vi "Main_01B.vi"() -> ()   [LabVIEW 2025]
uses:
  Utility/Universal Utility/TypeDefs_Utility/Cluster_Row-Column.ctl
  9e3f57c0-2ef8-4495-8287-c6a42a5fb955.vi
  Utility/Universal Utility/TypeDefs_Utility/ENUM_4 Directions U-D-L-R.ctl
  Utility/Universal Utility/TypeDefs_Utility/ENUM_8 Directions U-D-L-R.ctl
panel:
  out "count":i32[](array[numeric])
  out "positios":i32[](array[numeric])
  out "Direction Ticks":i32[](array[numeric])
  out "Array":bool[](array[boolean])
  out "MATCH":bool
  in  "Select Data":enum32{"Example", "Puzzle"}(tab)
  in  "Ex Answer":u32=6
  in  "Example":string="L68\nL30\nR48\nL5\nR60\nL55\nL1\nL99\nR14\nL82"
  in  "puzzel Answer":u32=7199
  in  "Puzzle":string="R46\nL11\nR26\nL29\nR14\nL26\nR18\nL38\nL48\nR45\nL8\nL48\nL2\nR34\nR4\nR8\nR35\nR41\nL16\nR31\nL36\nR16\nL22\nL35\nL33\nR42\nR42\nL43\nR28\nL31\nL38\nL47\nL29\nL13\nR13\nL17\nR16\nL20\nL16\nR18\nL21\nR41\nR37\nL10\nR48\nL44\nR26\nR17\nR7\nR78\nL90\nL33\nL91\nR74\nL56\nL53\nL90\nR97\nR42\nR30\nR17\nL47\nR4\nL4\nL23\nR23\nL66\nL45\nL82\nL23\nR90\nR70\nL29\nL66\nR51\nL54\nR54\nR32\nL48\nL95\nL57\nR63\nL14\nR86\nL67\nL45\nL39\nL35\nR19\nR19\nR45\nR87\nR89\nL83\nL57\nR22\nL22\nL36\nL53\nL95\nL616\nL87\nL13\nR67\nR933\nL70\nR75\nR74\nL16\nR20\nR17\nR45\nL92\nL64\nL61\nL28\nR541\nL42\nR1\nR27\nL77\nR850\nR39\nL39\nL373\nR66\nR53\nR16\nL28\nR66\nL7\nL68\nR355\nL80\nR52\nR48\nL16\nR13\nR78\nR330\nR995\nR57\nR643\nR31\nL26\nL1\nR96\nL93\nL48\nL59\nR..."
  out "Answer":u32
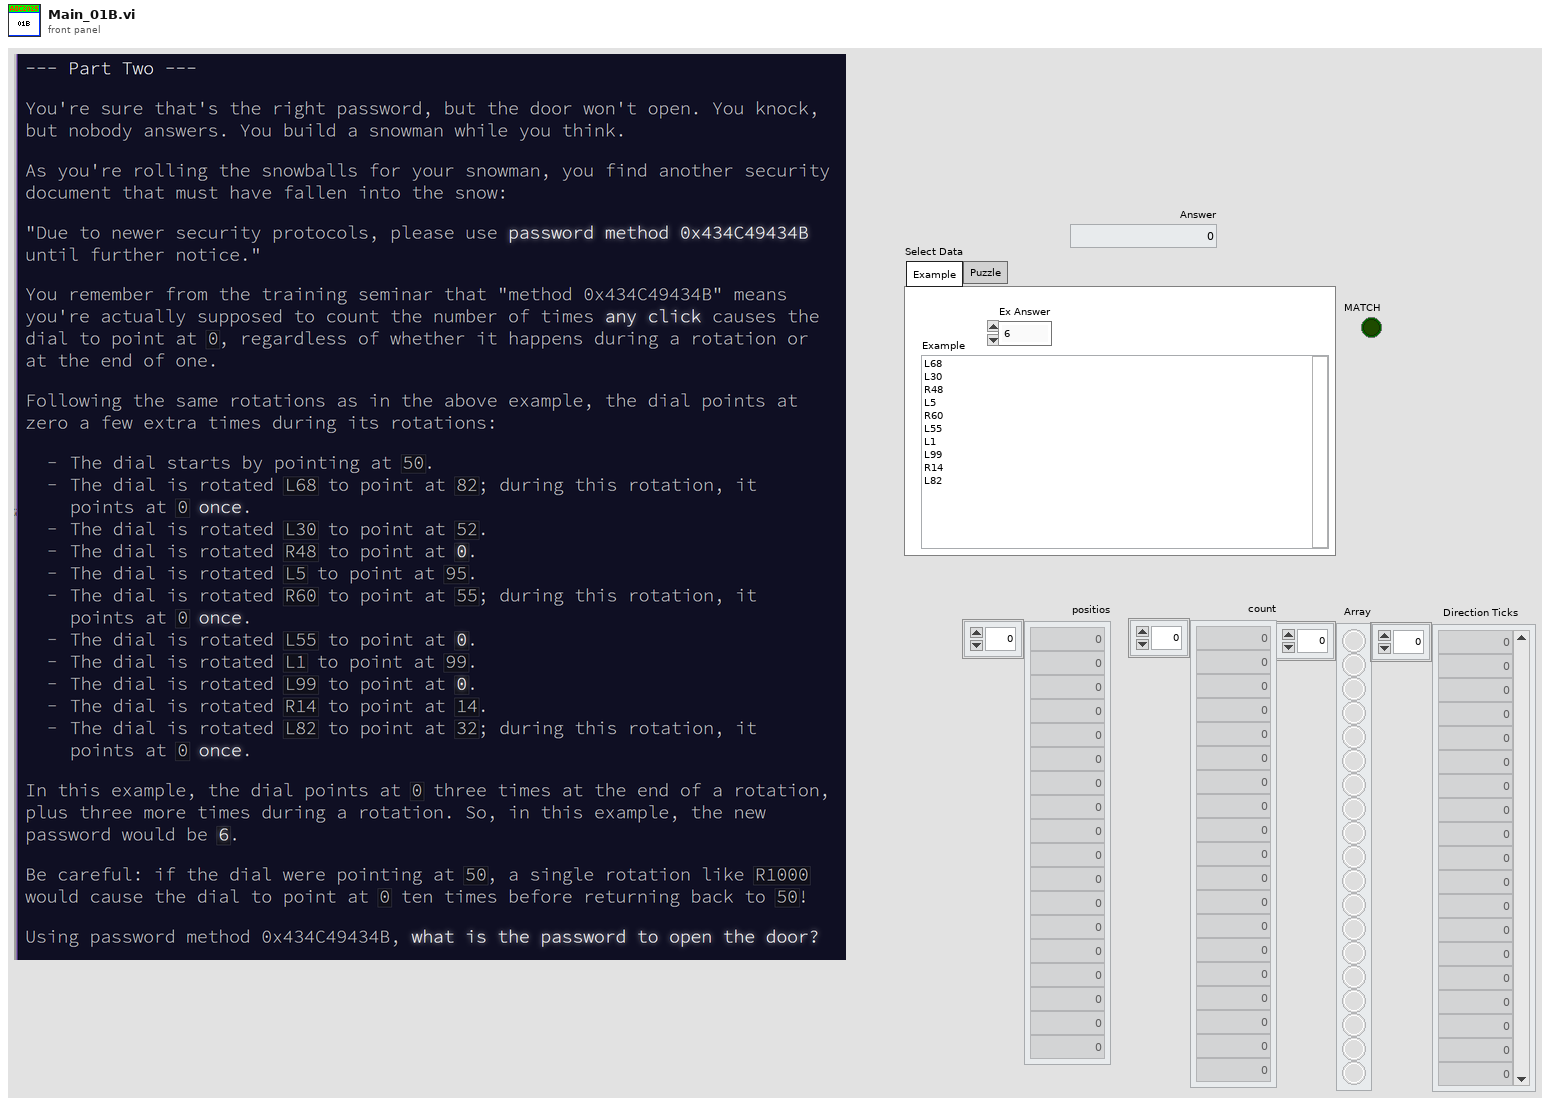
[diagram p1: front panel]
types:
  T1 = typedef "ENUM_8 Directions U-D-L-R.ctl" = enum16{"Up;-1,0", "Up-Right;-1,1", "Right;0,1", "Down-Right;1,1", "Down;1,0", "Down-Left;1,-1", "Left;0,-1", "Up-Left;-1,-1"}
  T2 = typedef "ENUM_4 Directions U-D-L-R.ctl" = enum16{"Up;-1,0", "Right;0,1", "Down;1,0", "Left;0,-1"}
  T3 = typedef "Cluster_Row-Column.ctl" = cluster{"R":i32, "C":i32}
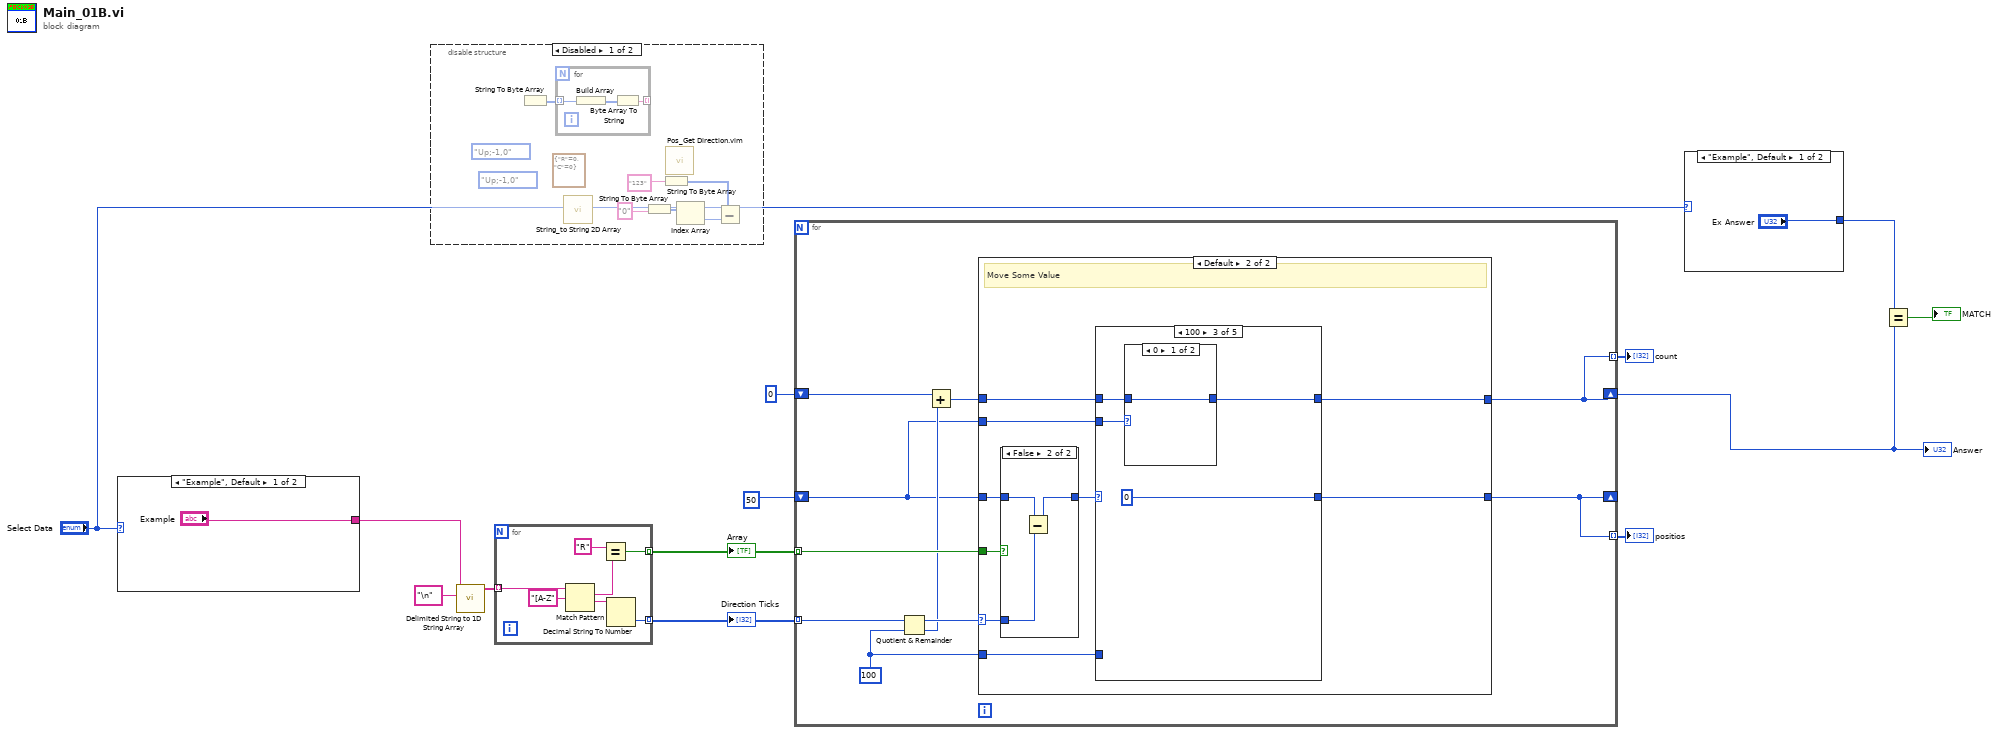
[diagram p0: block diagram]
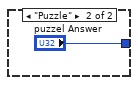
[diagram p2: hidden frame]
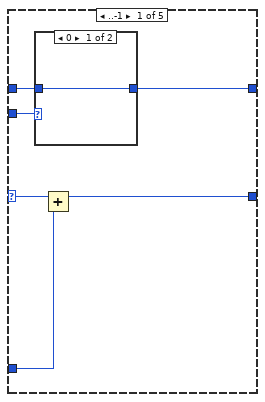
[diagram p4: hidden frame]
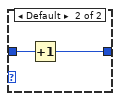
[diagram p5: hidden frame]
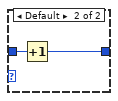
[diagram p7: hidden frame]
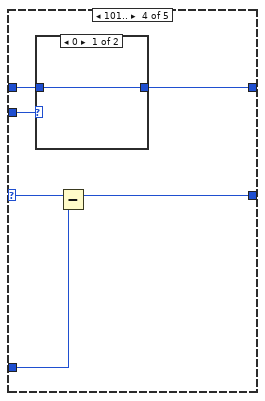
[diagram p8: hidden frame]
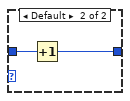
[diagram p9: hidden frame]
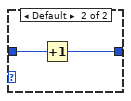
[diagram p11: hidden frame]
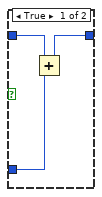
[diagram p12: hidden frame]
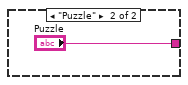
[diagram p13: hidden frame]
diagram:
  n1 = case shown="\"Example\", Default" "Select Data" {
    tunnel: ["Example" "Puzzle"] -> w11
    frame "Example", Default {
    }
    frame "Puzzle" {
    }
  }
  n2 = disable-structure shown="Disabled" {
    frame Disabled {
      (unwired) ENUM_8_Directions_U-D-L-R."Up;-1,0" ("Direction 8")
      (unwired) ENUM_4_Directions_U-D-L-R."Up;-1,0" ("Direction")
      (unwired) T3 {"R"=0, "C"=0} ("Position")
      n3 = String To Byte Array() -> (unsigned byte array=w16:u8[])  [unwired: 1 in]
      n4 = for {
        tunnel: w16 -> [w24] mode=indexing
        tunnel: [w22] -> _ mode=indexing
        n5 = Build Array(w24) -> (w23:u8[])
        n6 = Byte Array To String(unsigned byte array=w23) -> (string=w22:string)
      }
      n7 = call "String_to String 2D Array.vi"() -> ()  [unwired: 11 in, 1 out]
      n8 = String To Byte Array(string="0") -> (unsigned byte array=w19:u8[])
      n9 = String To Byte Array(string="123") -> (unsigned byte array=w17:u8[])
      n10 = call "Pos_Get Direction.vim"() -> ()  [unwired: 11 in, 1 out]
      n11 = Index Array(array=w19) -> (element=w18:u8)  [unwired: 1 in]
      n12 = Subtract(x=w17, y=w18) -> ()  [unwired: 1 out]
    }
    frame Enabled {
    }
  }
  n13 = call <vilib>:"Delimited String to 1D String Array.vi"("delimiter"="\n" ("delimiter (Tab)"), "delimited string"=w11) -> ("string array"=w12:string[])  [unwired: 9 in]
  n14 = for {
    tunnel: w12 -> [w31] mode=indexing
    tunnel: [w27] -> w9 mode=indexing
    tunnel: [w25] -> w8 mode=indexing
    n15 = Match Pattern(string=w31, regular expression="[A-Z") -> (match substring=w29:string, after substring=w26:string)  [unwired: 1 in, 2 out]
    n16 = Equal?(x="R", y=w29) -> (x = y?=w27:bool)
    n17 = Decimal String To Number(string=w26) -> (number=w25:i32)  [unwired: 2 in, 1 out]
  }
  "Array" <- w9
  "Direction Ticks" <- w8
  n18 = for {
    shift-right: [w38] -> _
    shift-left: 50 -> [w32]
    tunnel: w9 -> [w41] mode=indexing
    tunnel: w8 -> [w40] mode=indexing
    tunnel: [w38] -> w7 mode=indexing
    shift-right: [w37] -> w1
    shift-left: 0 -> [w39]
    tunnel: [w37] -> w2 mode=indexing
    w36 = 100 ("y")
    n19 = Quotient & Remainder(x=w40, y=w36) -> (x-y*floor(x/y)=w35:i32, floor(x/y)=w34:i32)
    n20 = Add(x=w39, y=w34) -> (x+y=w33:i32)
    n21 = case shown="Default" w35 {
      selector: w35 -> [_ w51]
      tunnel: w41 -> [_ w50]
      tunnel: w32 -> [w42 w52]
      tunnel: [w42 w45] -> w38
      tunnel: w36 -> [_ w46]
      tunnel: w33 -> [w43 w48]
      tunnel: [w43 w47] -> w37
      tunnel: w32 -> [_ w44]
      frame 0 {
        # "No More Movement"
      }
      frame Default {
        # "Move Some Value"
        n22 = case shown="False" w50 {
          tunnel: w52 -> [w89 w92]
          tunnel: w51 -> [w88 w91]
          tunnel: [w87 w90] -> w49
          frame True {
            n23 = Add(x=w89, y=w88) -> (x+y=w87:i32)
          }
          frame False {
            n24 = Subtract(x=w92, y=w91) -> (x-y=w90:i32)
          }
        }
        n25 = case shown="100" w49 {
          selector: w49 -> [w56 w62 _ w74 w81]
          tunnel: w48 -> [w58 w63 w67 w76 w83]
          tunnel: [w57 w63 w66 w75 w82] -> w47
          tunnel: w46 -> [w55 _ _ w73 _]
          tunnel: [w54 w62 0 w72 w81] -> w45
          tunnel: w44 -> [w53 _ w64 w71 w80]
          frame ..-1 {
            n26 = case shown="0" w53 {
              tunnel: w58 -> [w59 w61]
              tunnel: [w59 w60] -> w57
              frame 0 {
              }
              frame Default {
                n27 = Increment(x=w61) -> (x+1=w60:i32)
              }
            }
            n28 = Add(x=w56, y=w55) -> (x+y=w54:i32)
          }
          frame 1..99 {
          }
          frame 100 {
            n29 = case shown="0" w64 {
              tunnel: w67 -> [w68 w70]
              tunnel: [w68 w69] -> w66
              frame 0 {
              }
              frame Default {
                n30 = Increment(x=w70) -> (x+1=w69:i32)
              }
            }
          }
          frame 101.. {
            n31 = case shown="0" w71 {
              tunnel: w76 -> [w77 w79]
              tunnel: [w77 w78] -> w75
              frame 0 {
              }
              frame Default {
                n32 = Increment(x=w79) -> (x+1=w78:i32)
              }
            }
            n33 = Subtract(x=w74, y=w73) -> (x-y=w72:i32)
          }
          frame 0 {
            n34 = case shown="0" w80 {
              tunnel: w83 -> [w84 w86]
              tunnel: [w84 w85] -> w82
              frame 0 {
              }
              frame Default {
                n35 = Increment(x=w86) -> (x+1=w85:i32)
              }
            }
          }
        }
      }
    }
  }
  "Answer" <- w1
  "positios" <- w7
  "count" <- w2
  n36 = case shown="\"Example\", Default" "Select Data" {
    tunnel: ["Ex Answer" "puzzel Answer"] -> w5
    frame "Example", Default {
    }
    frame "Puzzle" {
    }
  }
  n37 = Equal?(x=w5, y=w1) -> (x = y?=→"MATCH":bool)
